vi "peirce_calcFactor.vi"(1 "n":i32 caption="ValoresDuvidosos", 2 "DesviosAbsolutos":dbl[](array[numeric])) -> (0 "x":dbl)   [LabVIEW 2016]
panel:
  in  "m":i32=1 caption="Variáveis"
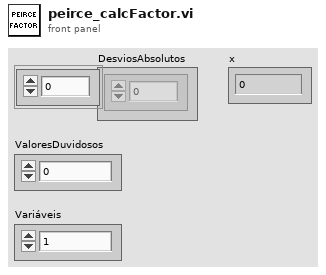
[diagram p1: front panel]
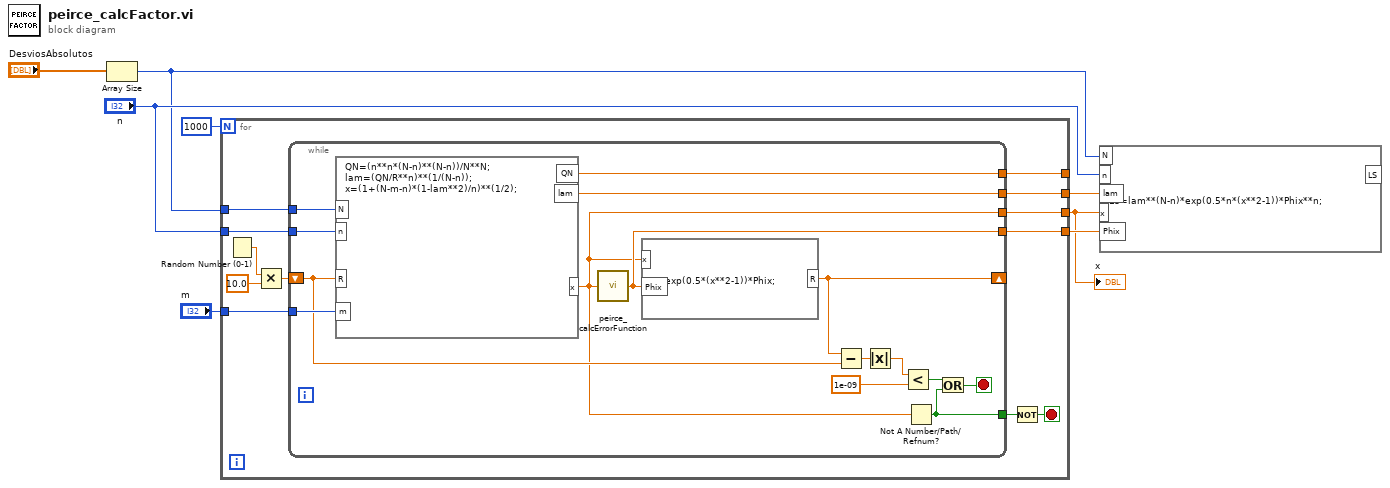
[diagram p0: block diagram]
diagram:
  n1 = Array Size(array="DesviosAbsolutos") -> (size(s)=w3:i32)
  n2 = for {
    N: 1000 -> [_]
    tunnel: "m" -> [w20]
    tunnel: w3 -> [w19]
    tunnel: "n" -> [w18]
    tunnel: [w17] -> w5
    tunnel: [w16] -> w1
    tunnel: [w15] -> w6
    tunnel: [w14] -> _
    stop <- w9 stop-if-true
    n3 = Random Number (0-1)() -> (number: 0 to 1=w12:dbl)
    n4 = Multiply(x=w12, y=10.0 ("input variable")) -> (x*y=w13:dbl)
    n5 = while {
      tunnel: w18 -> [w35]
      tunnel: w19 -> [w34]
      tunnel: w20 -> [w33]
      shift-right: [w29] -> _
      shift-left: w13 -> [w28]
      tunnel: [w27] -> w17
      tunnel: [w22] -> w16
      tunnel: [w26] -> w15
      tunnel: [w25] -> w14
      tunnel: [w21] -> w10
      stop <- w24 stop-if-true
      n6 = formula code="QN=(n**n*(N-n)**(N-n))/N**N;\nlam=(QN/R**n)**(1/(N-n));\nx=(1+(N-m-n)*(1-lam**2)/n)**(1/2);"("N"=w34, "n"=w35, "R"=w28, "m"=w33) -> ("QN"=w25:dbl, "x"=w22:dbl, "lam"=w27:dbl)
      n7 = call "peirce_calcErrorFunction.vi"("x"=w22) -> ("PhiX"=w26:dbl)
      n8 = formula code="R=exp(0.5*(x**2-1))*Phix;"("x"=w22, "Phix"=w26) -> ("R"=w29:dbl)
      n9 = Subtract(x=w29, y=w28) -> (x-y=w32:dbl)
      n10 = Absolute Value(x=w32) -> (abs(x)=w30:dbl)
      n11 = Less?(x=w30, y=1e-09) -> (x < y?=w23:bool)
      n12 = Not A Number/Path/Refnum?(number/path/refnum=w22) -> (NaN/Path/Refnum?=w21:bool)
      n13 = Or(x=w23, y=w21) -> (x .or. y?=w24:bool)
    }
    n14 = Not(x=w10) -> (.not. x?=w9:bool)
  }
  "x" <- w1
  n15 = formula code="LS=lam**(N-n)*exp(0.5*n*(x**2-1))*Phix**n;"("lam"=w5, "N"=w3, "n"="n", "x"=w1, "Phix"=w6) -> ()  [unwired: 1 out]
